vi "Ballard XML Generator.Open Label.vi"(0 "string in":string, 7 "input cluster":T1) -> (4 "string out":string)   [LabVIEW 2017]
uses:
  Controls/Database_Array.ctl
  Controls/Encoding.ctl
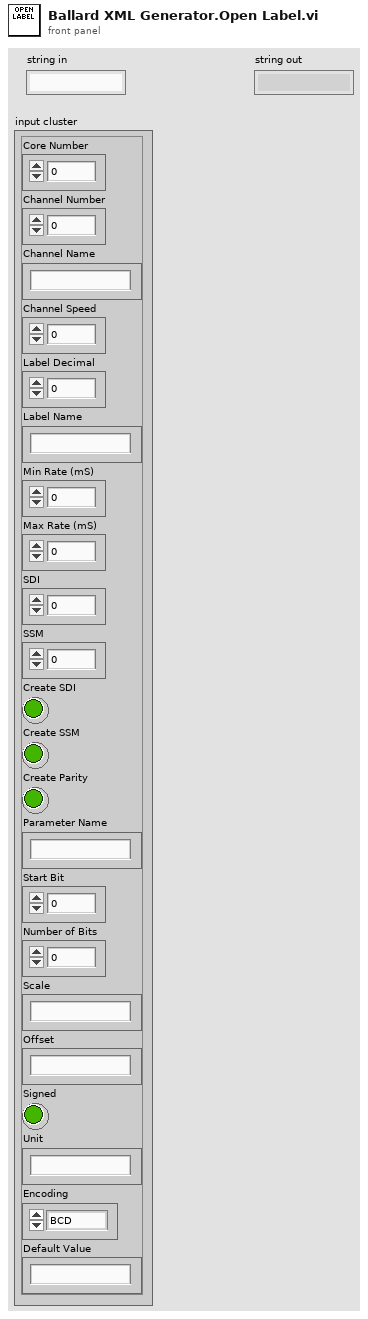
[diagram p1: front panel]
types:
  T1 = typedef "Database_Array.ctl" = cluster{"Core Number":i32, "Channel Number":i32, "Channel Name":string, "Channel Speed":i32, "Label Decimal":i32, "Label Name":string, "Min Rate (mS)":i32, "Max Rate (mS)":i32, "SDI":i32, "SSM":i32, "Create SDI":bool, "Create SSM":bool, "Create Parity":bool, "Parameter Name":string, "Start Bit":i32, "Number of Bits":i32, "Scale":string, "Offset":string, "Signed":bool, "Unit":string, "Encoding":T2, "Default Value":string}
  T2 = typedef "Encoding.ctl" = enum16{"BCD", "BNR", "Discrete"}
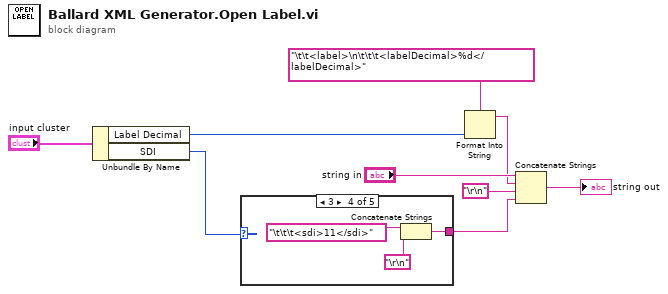
[diagram p0: block diagram]
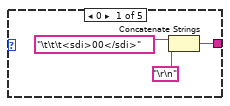
[diagram p2: hidden frame]
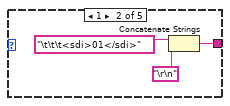
[diagram p3: hidden frame]
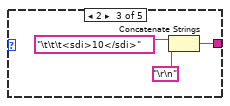
[diagram p4: hidden frame]
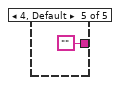
[diagram p5: hidden frame]
diagram:
  n1 = Unbundle By Name("input cluster") -> ("Label Decimal"=w2:i32, "SDI"=w1:i32)
  n2 = case shown="3" w1 {
    tunnel: [w11 w14 w17 w20 ""] -> w5
    frame 0 {
      n3 = Concatenate Strings("\t\t\t<sdi>00</sdi>", "\r\n") -> (w11:string)
    }
    frame 1 {
      n4 = Concatenate Strings("\t\t\t<sdi>01</sdi>", "\r\n") -> (w14:string)
    }
    frame 2 {
      n5 = Concatenate Strings("\t\t\t<sdi>10</sdi>", "\r\n") -> (w17:string)
    }
    frame 3 {
      n6 = Concatenate Strings("\t\t\t<sdi>11</sdi>", "\r\n") -> (w20:string)
    }
    frame 4, Default {
    }
  }
  n7 = Format Into String(format string="\t\t<label>\n\t\t\t<labelDecimal>%d</labelDecimal>", w2) -> (resulting string=w6:string)  [unwired: 2 in, 1 out]
  n8 = Concatenate Strings("string in", w6, "\r\n", w5) -> (→"string out":string)
